vi "get data definition.vi"(10 "channel classification":T1, 11 "GPIC Core runtime in":refnum<class "GPIC Core runtime.lvclass">) -> (1 "valid?":bool, 2 "index cluster":variant, 3 "GPIC Core runtime out":refnum<class "GPIC Core runtime.lvclass">)   [LabVIEW 2017, in "GPIC Core runtime.lvclass"]
uses:
  GPIC Core runtime.lvclass
  <vilib>/NI/Tag Bus Module Framework/channel/channel classification.ctl
  input user data.ctl
  output user data.ctl
  parameter user data.ctl
  result user data.ctl
  <vilib>/NI/Tag Bus Module Framework/channel/TBM channel.lvclass
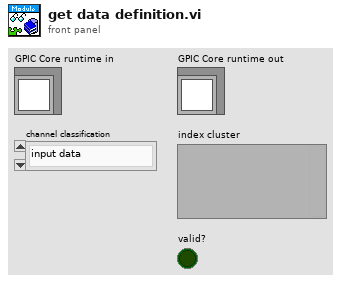
[diagram p1: front panel]
types:
  T1 = typedef "TBM channel.lvclass/channel classification.ctl" = enum16{"input data", "output data", "processing parameter", "processing result"}
  T2 = typedef "GPIC Core runtime.lvclass/input user data.ctl" = cluster{"AO_AO0":i16, "AO_AO1":i16, "AO_AO2":i16, "AO_AO3":i16, "AO_AO4":i16, "AO_AO5":i16, "AO_AO6":i16, "AO_AO7":i16, "HalfBridge_DO0":bool, "HalfBridge_DO1":bool, "HalfBridge_DO2":bool, "HalfBridge_DO3":bool, "HalfBridge_DO4":bool, "HalfBridge_DO5":bool, "HalfBridge_DO6":bool, "HalfBridge_DO7":bool, "HalfBridge_DO8":bool, "HalfBridge_DO9":bool, "HalfBridge_DO10":bool, "HalfBridge_DO11":bool, "HalfBridge_DO12":bool, "HalfBridge_DO13":bool, "LVTTL_DIO0":bool, "LVTTL_DIO1":bool, "LVTTL_DIO2":bool, "LVTTL_DIO3":bool, "LVTTL_DIO4":bool, "LVTTL_DIO5":bool, "LVTTL_DIO6":bool, "LVTTL_DIO7":bool, "LVTTL_DIO8":bool, "LVTTL_DIO9":bool, "LVTTL_DIO10":bool, "LVTTL_DIO11":bool, "LVTTL_DIO12":bool, "LVTTL_DIO13":bool, "LVTTL_DIO14":bool, "LVTTL_DIO15":bool, "LVTTL_DIO16":bool, "LVTTL_DIO17":bool, "LVTTL_DIO18":bool, "LVTTL_DIO19":bool, "LVTTL_DIO20":bool, "LVTTL_DIO21":bool, "LVTTL_DIO22":bool, "LVTTL_DIO23":bool, "LVTTL_DIO24":bool, "LVTTL_DIO25":bool, "LVTTL_DIO26":bool, "LVTTL_DIO27":bool, "LVTTL_DIO28":bool, "LVTTL_DIO29":bool, "LVTTL_DIO30":bool, "LVTTL_DIO31":bool, "RelayControl_DO0":bool, "RelayControl_DO1":bool, "RelayContro_DOl2":bool, "RelayControl_DO3":bool, "Scanned_AI0":sgl, "Scanned_AI1":sgl, "Scanned_AI2":sgl, "Scanned_AI3":sgl, "Scanned_AI4":sgl, "Scanned_AI5":sgl, "Scanned_AI6":sgl, "Scanned_AI7":sgl, "Simultaneous_AI0":sgl, "Simultaneous_AI1":sgl, "Simultaneous_AI2":sgl, "Simultaneous_AI3":sgl, "Simultaneous_AI4":sgl, "Simultaneous_AI5":sgl, "Simultaneous_AI6":sgl, "Simultaneous_AI7":sgl, "Simultaneous_AI8":sgl, "Simultaneous_AI9":sgl, "Simultaneous_AI10":sgl, "Simultaneous_AI11":sgl, "Simultaneous_AI12":sgl, "Simultaneous_AI13":sgl, "Simultaneous_AI14":sgl, "Simultaneous_AI15":sgl, "Sinking_DO0":bool, "Sinking_DO1":bool, "Sinking_DO2":bool, "Sinking_DO3":bool, "Sinking_DO4":bool, "Sinking_DO5":bool, "Sinking_DO6":bool, "Sinking_DO7":bool, "Sinking_DO8":bool, "Sinking_DO9":bool, "Sinking_DO10":bool, "Sinking_DO11":bool, "Sinking_DO12":bool, "Sinking_DO13":bool, "Sinking_DO14":bool, "Sinking_DO15":bool, "Sinking_DO16":bool, "Sinking_DO17":bool, "Sinking_DO18":bool, "Sinking_DO19":bool, "Sinking_DO20":bool, "Sinking_DO21":bool, "Sinking_DO22":bool, "Sinking_DO23":bool, "Sourcing_P0_DI0":bool, "Sourcing_P0_DI1":bool, "Sourcing_P0_DI2":bool, "Sourcing_P0_DI3":bool, "Sourcing_P0_DI4":bool, "Sourcing_P0_DI5":bool, "Sourcing_P0_DI6":bool, "Sourcing_P0_DI7":bool, "Sourcing_P0_DI8":bool, "Sourcing_P0_DI9":bool, "Sourcing_P0_DI10":bool, "Sourcing_P0_DI11":bool, "Sourcing_P0_DI12":bool, "Sourcing_P0_DI13":bool, "Sourcing_P1_DI0":bool, "Sourcing_P1_DI1":bool, "Sourcing_P1_DI2":bool, "Sourcing_P1_DI3":bool, "Sourcing_P1_DI4":bool, "Sourcing_P1_DI5":bool, "Sourcing_P1_DI6":bool, "Sourcing_P1_DI7":bool, "Sourcing_P1_DI8":bool, "Sourcing_P1_DI9":bool, "Sourcing_P1_DI10":bool, "Sourcing_P1_DI11":bool, "Sourcing_P1_DI12":bool, "Sourcing_P1_DI13":bool}
  T3 = typedef "GPIC Core runtime.lvclass/output user data.ctl" = cluster{"fmwk_placeholder":i32}
  T4 = typedef "GPIC Core runtime.lvclass/parameter user data.ctl" = cluster{"fmwk_placeholder":i32}
  T5 = typedef "GPIC Core runtime.lvclass/result user data.ctl" = cluster{"fmwk_placeholder":i32}
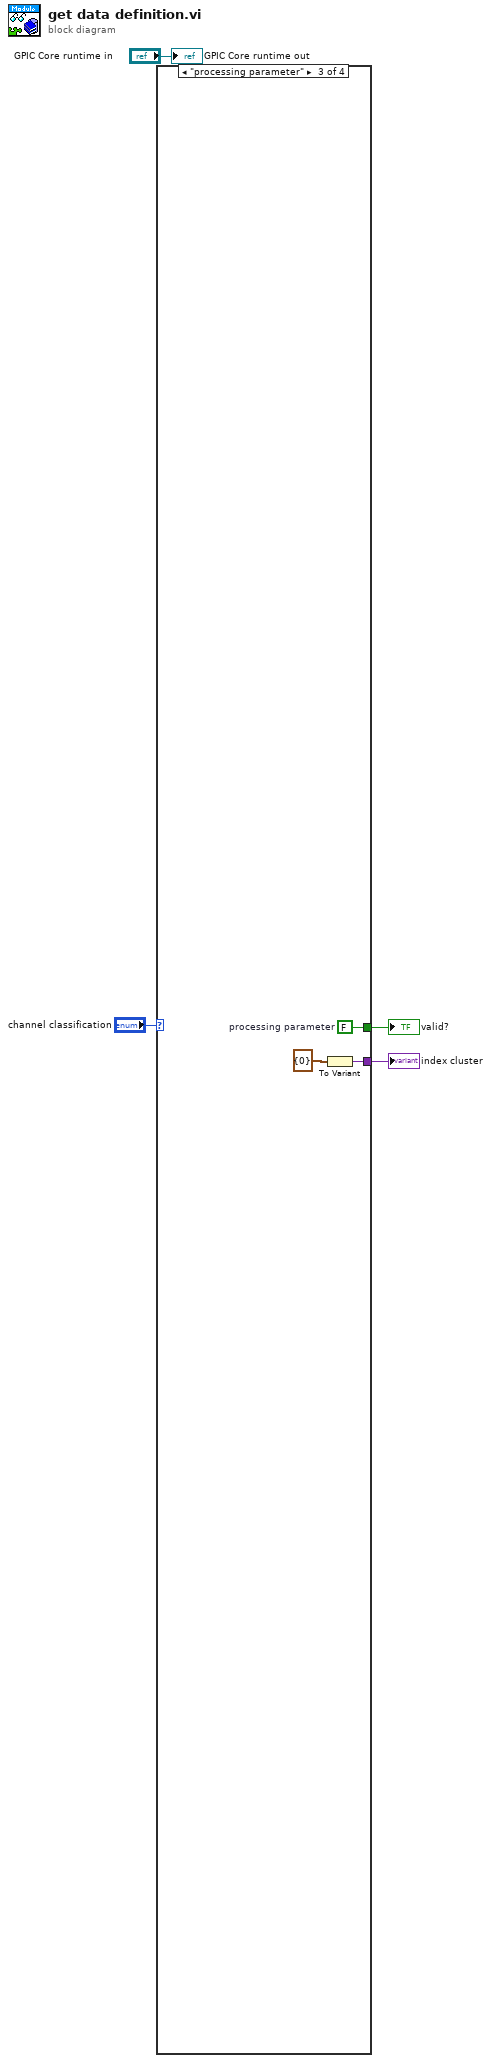
[diagram p0: block diagram]
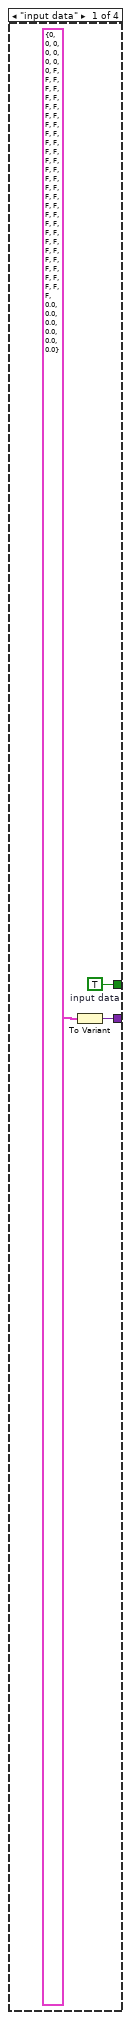
[diagram p2: hidden frame]
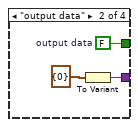
[diagram p3: hidden frame]
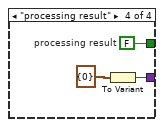
[diagram p4: hidden frame]
diagram:
  n1 = case shown="\"processing parameter\"" "channel classification" {
    tunnel: [w6 w10 w13 w16] -> w2
    tunnel: [w5 w9 w12 w15] -> w1
    frame "input data" {
      w5 = TRUE  # input data
      n2 = To Variant(anything=T2 {"AO_AO0"=0, "AO_AO1"=0, "AO_AO2"=0, "AO_AO3"=0, "AO_AO4"=0, "AO_AO5"=0, "AO_AO6"=0, "AO_AO7"=0, "HalfBridge_DO0"=FALSE, "HalfBridge_DO1"=FALSE, "HalfBridge_DO2"=FALSE, "HalfBridge_DO3"=FALSE, "HalfBridge_DO4"=FALSE, "HalfBridge_DO5"=FALSE, "HalfBridge_DO6"=FALSE, "HalfBridge_DO7"=FALSE, "HalfBridge_DO8"=FALSE, "HalfBridge_DO9"=FALSE, "HalfBridge_DO10"=FALSE, "HalfBridge_DO11"=FALSE, "HalfBridge_DO12"=FALSE, "HalfBridge_DO13"=FALSE, "LVTTL_DIO0"=FALSE, "LVTTL_DIO1"=FALSE, "LVTTL_DIO2"=FALSE, "LVTTL_DIO3"=FALSE, "LVTTL_DIO4"=FALSE, "LVTTL_DIO5"=FALSE, "LVTTL_DIO6"=FALSE, "LVTTL_DIO7"=FALSE, "LVTTL_DIO8"=FALSE, "LVTTL_DIO9"=FALSE, "LVTTL_DIO10"=FALSE, "LVTTL_DIO11"=FALSE, "LVTTL_DIO12"=FALSE, "LVTTL_DIO13"=FALSE, "LVTTL_DIO14"=FALSE, "LVTTL_DIO15"=FALSE, "LVTTL_DIO16"=FALSE, "LVTTL_DIO17"=FALSE, "LVTTL_DIO18"=FALSE, "LVTTL_DIO19"=FALSE, "LVTTL_DIO20"=FALSE, "LVTTL_DIO21"=FALSE, "LVTTL_DIO22"=FALSE, "LVTTL_DIO23"=FALSE, "LVTTL_DIO24"=FALSE, "LVTTL_DIO25"=FALSE, "LVTTL_DIO26"=FALSE, "LVTTL_DIO27"=FALSE, "LVTTL_DIO28"=FALSE, "LVTTL_DIO29"=FALSE, "LVTTL_DIO30"=FALSE, "LVTTL_DIO31"=FALSE, "RelayControl_DO0"=FALSE, "RelayControl_DO1"=FALSE, "RelayContro_DOl2"=FALSE, "RelayControl_DO3"=FALSE, "Scanned_AI0"=0.0, "Scanned_AI1"=0.0, "Scanned_AI2"=0.0, "Scanned_AI3"=0.0, "Scanned_AI4"=0.0, "Scanned_AI5"=0.0, "Scanned_AI6"=0.0, "Scanned_AI7"=0.0, "Simultaneous_AI0"=0.0, "Simultaneous_AI1"=0.0, "Simultaneous_AI2"=0.0, "Simultaneous_AI3"=0.0, "Simultaneous_AI4"=0.0, "Simultaneous_AI5"=0.0, "Simultaneous_AI6"=0.0, "Simultaneous_AI7"=0.0, "Simultaneous_AI8"=0.0, "Simultaneous_AI9"=0.0, "Simultaneous_AI10"=0.0, "Simultaneous_AI11"=0.0, "Simultaneous_AI12"=0.0, "Simultaneous_AI13"=0.0, "Simultaneous_AI14"=0.0, "Simultaneous_AI15"=0.0, "Sinking_DO0"=FALSE, "Sinking_DO1"=FALSE, "Sinking_DO2"=FALSE, "Sinking_DO3"=FALSE, "Sinking_DO4"=FALSE, "Sinking_DO5"=FALSE, "Sinking_DO6"=FALSE, "Sinking_DO7"=FALSE, "Sinking_DO8"=FALSE, "Sinking_DO9"=FALSE, "Sinking_DO10"=FALSE, "Sinking_DO11"=FALSE, "Sinking_DO12"=FALSE, "Sinking_DO13"=FALSE, "Sinking_DO14"=FALSE, "Sinking_DO15"=FALSE, "Sinking_DO16"=FALSE, "Sinking_DO17"=FALSE, "Sinking_DO18"=FALSE, "Sinking_DO19"=FALSE, "Sinking_DO20"=FALSE, "Sinking_DO21"=FALSE, "Sinking_DO22"=FALSE, "Sinking_DO23"=FALSE, "Sourcing_P0_DI0"=FALSE, "Sourcing_P0_DI1"=FALSE, "Sourcing_P0_DI2"=FALSE, "Sourcing_P0_DI3"=FALSE, "Sourcing_P0_DI4"=FALSE, "Sourcing_P0_DI5"=FALSE, "Sourcing_P0_DI6"=FALSE, "Sourcing_P0_DI7"=FALSE, "Sourcing_P0_DI8"=FALSE, "Sourcing_P0_DI9"=FALSE, "Sourcing_P0_DI10"=FALSE, "Sourcing_P0_DI11"=FALSE, "Sourcing_P0_DI12"=FALSE, "Sourcing_P0_DI13"=FALSE, "Sourcing_P1_DI0"=FALSE, "Sourcing_P1_DI1"=FALSE, "Sourcing_P1_DI2"=FALSE, "Sourcing_P1_DI3"=FALSE, "Sourcing_P1_DI4"=FALSE, "Sourcing_P1_DI5"=FALSE, "Sourcing_P1_DI6"=FALSE, "Sourcing_P1_DI7"=FALSE, "Sourcing_P1_DI8"=FALSE, "Sourcing_P1_DI9"=FALSE, "Sourcing_P1_DI10"=FALSE, "Sourcing_P1_DI11"=FALSE, "Sourcing_P1_DI12"=FALSE, "Sourcing_P1_DI13"=FALSE} ("Inputs from system")) -> (Variant=w6:variant)
    }
    frame "output data" {
      w9 = FALSE  # output data
      n3 = To Variant(anything=T3 {"fmwk_placeholder"=0} ("Outputs to system")) -> (Variant=w10:variant)
    }
    frame "processing parameter" {
      w12 = FALSE  # processing parameter
      n4 = To Variant(anything=T4 {"fmwk_placeholder"=0} ("Parameters to process")) -> (Variant=w13:variant)
    }
    frame "processing result" {
      w15 = FALSE  # processing result
      n5 = To Variant(anything=T5 {"fmwk_placeholder"=0} ("Results from processing")) -> (Variant=w16:variant)
    }
  }
  "index cluster" <- w2
  "valid?" <- w1
  "GPIC Core runtime out" <- "GPIC Core runtime in"
